vi "Start Logging.vi"(8 "error in (no error)":errorcluster, 9 "Actor to Log":refnum<class "Message Enqueuer.lvclass">, 10 "Label":string, 11 "Classic Logger in":refnum<class "Classic Logger.lvclass">) -> (0 "error out":errorcluster, 3 "Classic Logger out":refnum<class "Classic Logger.lvclass">)   [LabVIEW 2017, in "MGI-Monitored Actor.lvlib" / "Classic Logger.lvclass"]
uses:
  Classic Logger.lvclass
  <vilib>/ActorFramework/Message Enqueuer/Message Enqueuer.lvclass
  Classic Logger.lvclass/Classic Logger.ctl
  monitored-actor-core/Source/Monitored Actor/Monitored Actor Messages/Enable Message Logging Msg/Enable Message Logging Msg.lvclass
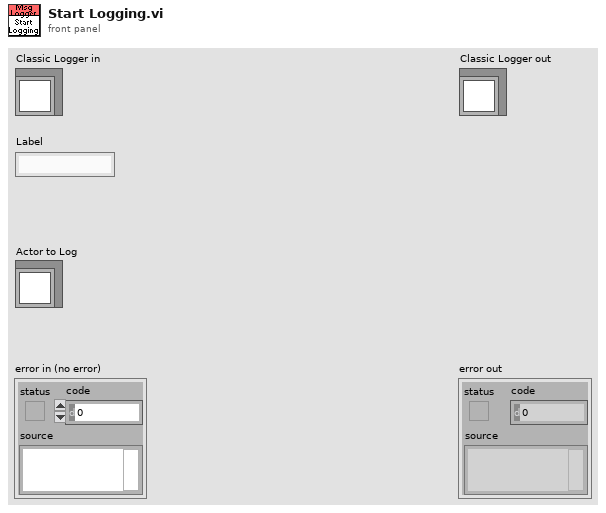
[diagram p1: front panel]
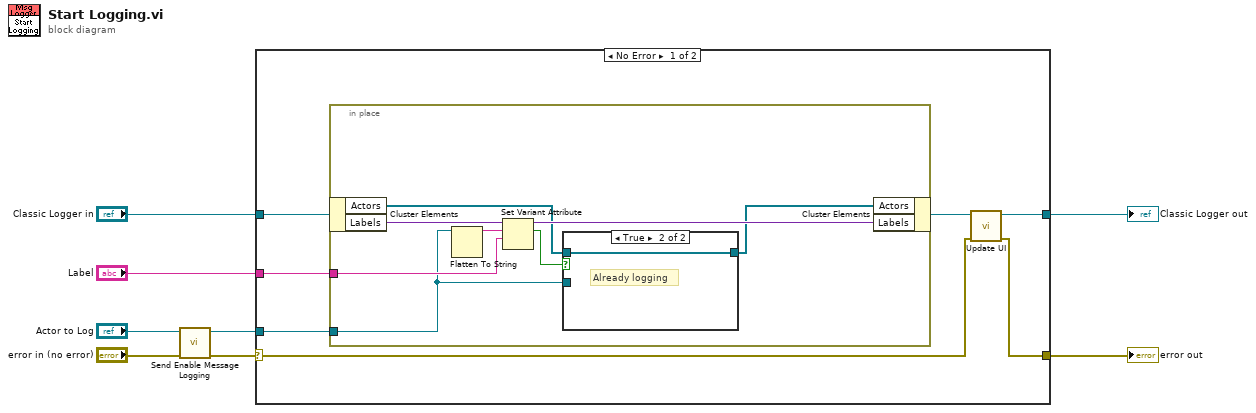
[diagram p0: block diagram]
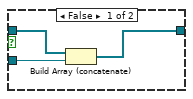
[diagram p2: hidden frame]
diagram:
  n1 = call "Send Enable Message Logging.vi"("error in (no error)"="error in (no error)", "Message Enqueuer in"="Actor to Log") -> ("error out"=w2:errorcluster, "Message Enqueuer out"=w4:refnum<class "Message Enqueuer.lvclass">)  [unwired: 8 in]
  n2 = case shown="No Error" w2 {
    selector: w2 -> [w10 w28]
    tunnel: "Classic Logger in" -> [w15 w29]
    tunnel: [w11 w29] -> w7
    tunnel: "Label" -> [w13 _]
    tunnel: w4 -> [w12 _]
    tunnel: [w9 w28] -> w1
    frame No Error {
      n3 = in-place {
        in-place-border: w13 -> [w21]
        in-place-border: w12 -> [w17]
        n4 = in-place-cluster #1(w15) -> ("Actors"=w19:refnum<class "Message Enqueuer.lvclass">[], "Labels"=w23:variant)
        n5 = Flatten To String(anything=w17) -> (data string=w22:string)  [unwired: 3 in, 2 out]
        n6 = Set Variant Attribute(Variant=w23, name=w22, value=w21) -> (Variant out=w20:variant, replaced=w16:bool)  [unwired: 1 in, 1 out]
        n7 = case shown="True" w16 {
          tunnel: w19 -> [w26 w27]
          tunnel: [w25 w27] -> w18
          tunnel: w17 -> [w24 _]
          frame False {
            n8 = Build Array (concatenate)(w26, w24) -> (w25:refnum<class "Message Enqueuer.lvclass">[])
          }
          frame True {
            # "Already logging"
          }
        }
        n9 = in-place-cluster #1("Actors"=w18, "Labels"=w20) -> (w14:refnum<class "Classic Logger.lvclass">)
      }
      n10 = call "Update UI.vi"("error in (no error)"=w10, "Message Logger in"=w14) -> ("error out"=w9:errorcluster, "Message Logger out"=w11:refnum<class "Classic Logger.lvclass">)  [unwired: 8 in]
    }
    frame Error {
    }
  }
  "error out" <- w1
  "Classic Logger out" <- w7
